vi "Read Element of Thrust Allocation Matrix.vi"(8 "error in (no error)":errorcluster, 10 "indices":i32[](array[numeric]), 11 "Thrust Allocation in":refnum<class "Thrust Allocation.lvclass">) -> (0 "error out":errorcluster, 2 "Real Matrix Element":dbl, 3 "Thrust Allocation out":refnum<class "Thrust Allocation.lvclass">)   [LabVIEW 2014, in "Thrust Allocation.lvclass"]
uses:
  Thrust Allocation.lvclass
  Thrust Allocation.lvclass/Thrust Allocation.ctl
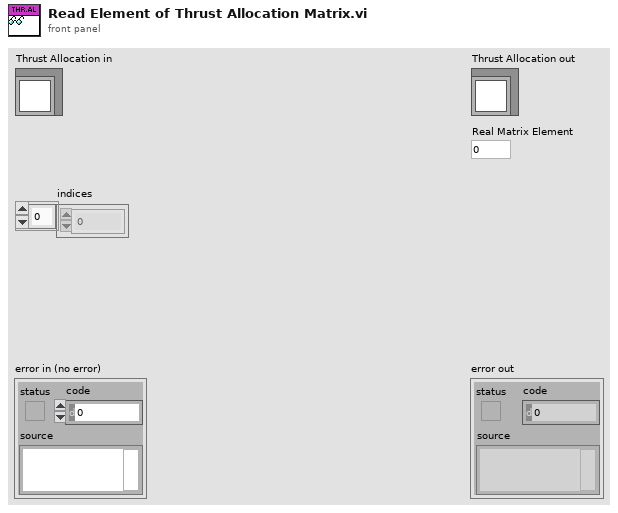
[diagram p1: front panel]
types:
  T1 = typedef "NI_Matrix.lvlib/RealMatrix.ctl" = dbl[][]
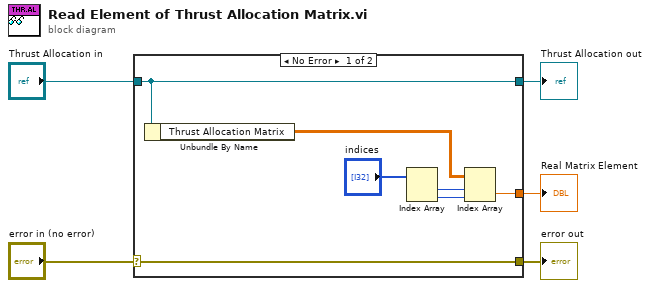
[diagram p0: block diagram]
diagram:
  n1 = case shown="No Error" "error in (no error)" {
    selector: "error in (no error)" -> [w12 w13]
    tunnel: [w12 w13] -> w4
    tunnel: [w11 w14] -> w2
    tunnel: "Thrust Allocation in" -> [w11 w14]
    tunnel: [w10 _] -> w1
    frame No Error {
      n2 = Unbundle By Name(w11) -> ("Thrust Allocation Matrix"=w6:T1)
      n3 = Index Array(array="indices") -> (element #1=w8:i32, element #2=w7:i32)  [unwired: 2 in]
      n4 = Index Array(array=w6, index (row)=w8, index (col)=w7) -> (element=w10:dbl)
    }
    frame Error {
    }
  }
  "error out" <- w4
  "Thrust Allocation out" <- w2
  "Real Matrix Element" <- w1
